vi "ReadFile.vi"(8 "error in":errorcluster, 10 "section":string="Script", 11 "file path (use dialog)":path) -> (0 "error out":errorcluster, 2 "found?":bool, 3 "Commands Sent To SSM":string[](array[string])=["AcPwrInit", "AcPwrConfig", "AcPwrStartMeas,PPS,1", "AcPwrStartMeas,Chroma", "AcPwrDeviceOn,Chroma", "Delay,2000", "AcPwrDeviceOff,Chroma", "Delay,2000", "AcPwrDeviceOn,Chroma", "Delay,2000", "AcPwrDeviceOff,Chroma", "Delay,2000", "AcPwrDeviceOn,PPS", "AcPwrDeviceOff,PPS", "AcPwrClose,PPS", "AcPwrClose,Chroma", "Stop"])   [LabVIEW 2018, in "Test.lvclass"]
doc: "Reads an array of string commands from a provided ini file. The section input details which portion of the file should be read."
uses:
  Test.lvclass
  <vilib>/Utility/config.llb/NI_LVConfig.lvlib
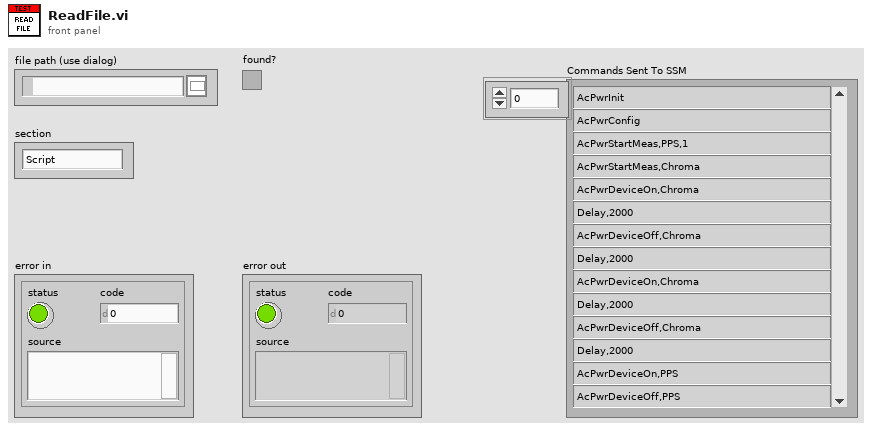
[diagram p1: front panel]
types:
  T1 = typedef "NI_LVConfig.lvlib/Config Data RefNum.ctl" = refnum<k1>
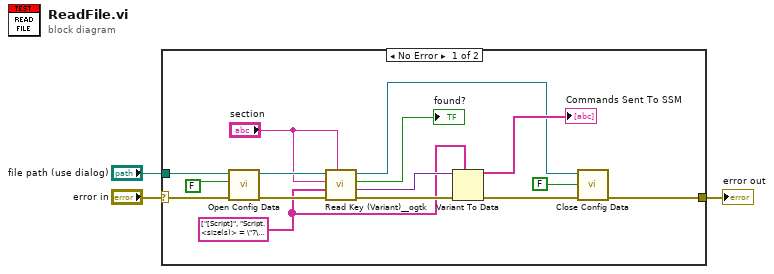
[diagram p0: block diagram]
diagram:
  n1 = case shown="No Error" "error in" {
    selector: "error in" -> [w12 w19]
    tunnel: [w6 w19] -> w2
    tunnel: "file path (use dialog)" -> [w5 _]
    frame No Error {
      w4 = string[] ["[Script]", "Script.<size(s)> = \"7\"", "Script 0 = \"ErrorSeverity,Abort\"", "Script 1 = \"SensorCreateSession,SiemensDEM0\"", "Script 2 = \"SensorConfig,SiemensDEM0\"", "Script 3 = \"SensorStart,SiemensDEM0\"", "Script 4 = \"Delay,5000\"", "Script 5 = \"SensorStop,SiemensDEM0\""] ("Commands Sent To SSM")
      n2 = call <vilib>:"Open Config Data.vi"("error in (no error)"=w12, "create file if necessary (T)"=FALSE, "configuration file path"=w5) -> ("error out"=w16:errorcluster, "refnum"=w17:T1)  [unwired: 6 in, 1 out]
      n3 = call <userlib>:"Read Key (Variant)__ogtk.vi"("section"="section", "error in (no error)"=w16, "type"=w4, "key (optional)"="section", "refnum"=w17) -> ("error out"=w14:errorcluster, "key-value"=w15:variant, "found?"=→"found?":bool, "refnum out"=w7:T1)  [unwired: 3 in]
      n4 = Variant To Data(error in=w14, type=w4, Variant=w15) -> (data=→"Commands Sent To SSM":string[], error out=w8:errorcluster)
      n5 = call <vilib>:"Close Config Data.vi"("error in (no error)"=w8, "write file if changed (T)"=FALSE, "refnum"=w7) -> ("error out"=w6:errorcluster)  [unwired: 7 in, 1 out]
    }
    frame Error {
    }
  }
  "error out" <- w2
